vi "saveDataNodeBegin.vi"(8 "error in (no error)":errorcluster, 9 "indent":i32, 10 "XML Refnum in":refnum<file>, 11 "Channel in":refnum<class "Channel.lvclass">) -> (0 "error out":errorcluster, 2 "XML Refnum out":refnum<file>, 3 "Chennel out":refnum<class "Channel.lvclass">)   [LabVIEW 2014, in "Channel.lvclass"]
doc: "Begins the process of saving a xceData Node to an XML formatted file."
uses:
  Channel.lvclass
  Channel.lvclass/Channel.ctl
  xCE/xceDataNode/xceDataNode.lvclass
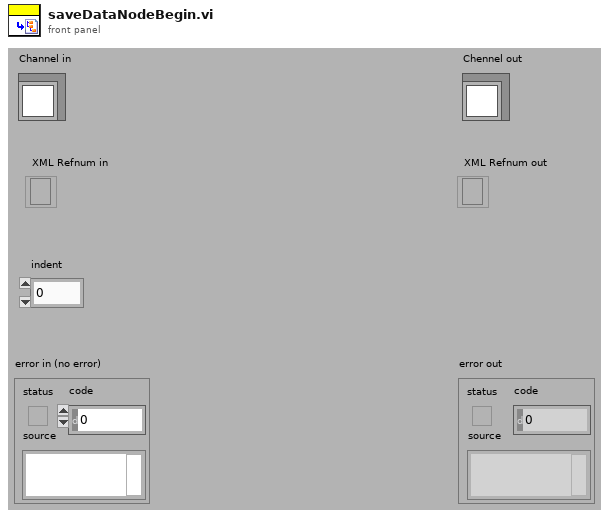
[diagram p1: front panel]
types:
  T1 = typedef "enum_Symbols.ctl" = enum16{"Default", "Analog Input", "Analog Output", "Digital Input", "Digital Output", "PWM Input", "PWM Output"}
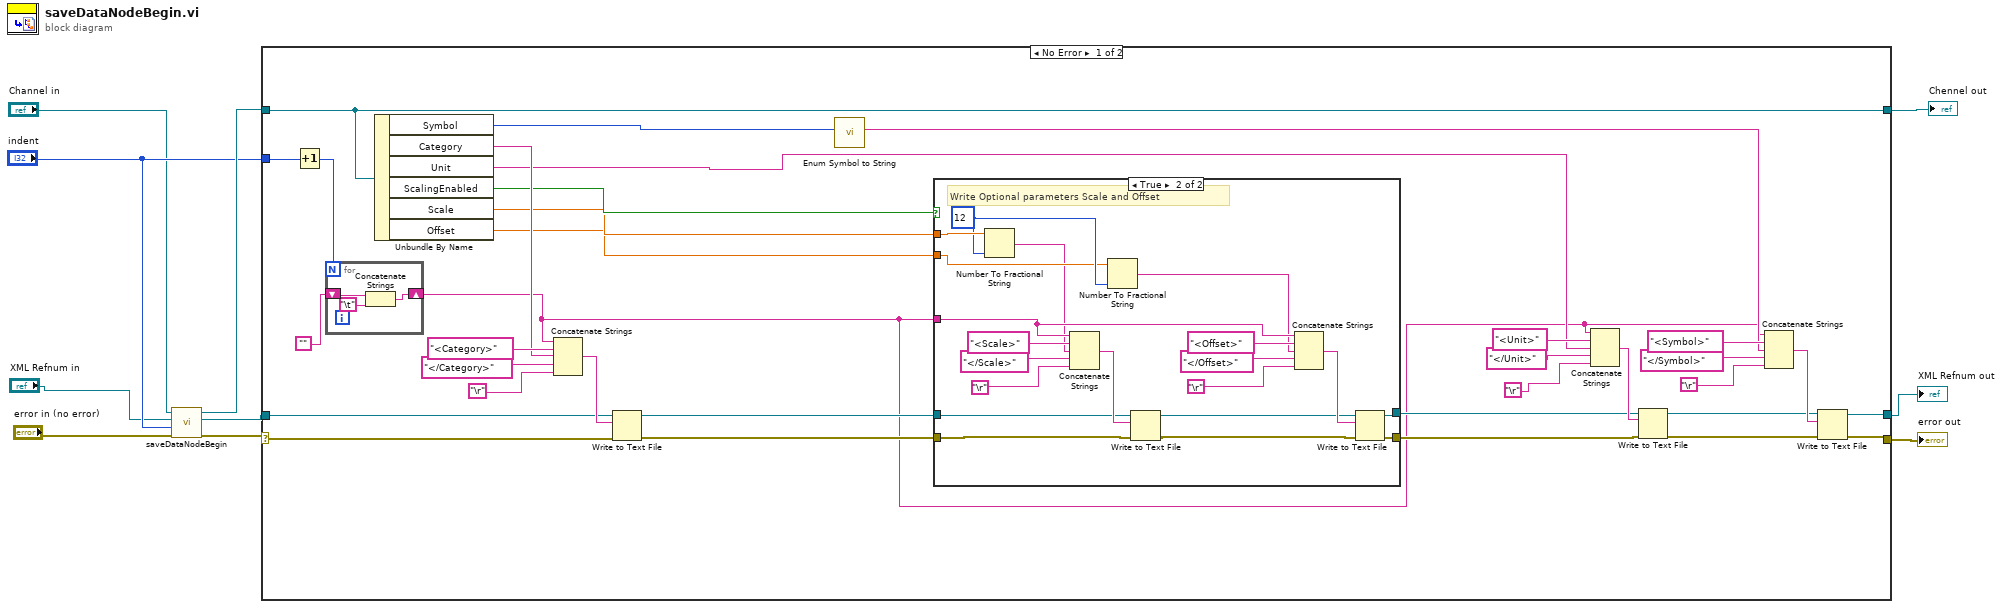
[diagram p0: block diagram]
diagram:
  n1 = call-parent "saveDataNodeBegin.vi"("error in (no error)"="error in (no error)", "indent"="indent", "XML Refnum in"="XML Refnum in", "xceDataNode in"="Channel in") -> ("error out"=w6:errorcluster, "XML Refnum out"=w5:refnum<file>, "xceDataNode out"=w4:refnum<class "Channel.lvclass">)  [unwired: 5 in]
  n2 = case shown="No Error" w6 {
    selector: w6 -> [w33 w71]
    tunnel: w4 -> [w35 w72]
    tunnel: [w35 w72] -> w10
    tunnel: [w12 w71] -> w8
    tunnel: [w13 w70] -> w9
    tunnel: "indent" -> [w36 _]
    tunnel: w5 -> [w34 w70]
    frame No Error {
      n3 = Increment(x=w36) -> (x+1=w43:i32)
      n4 = for {
        N: w43 -> [_]
        shift-right: [w67] -> w11
        shift-left: "" -> [w69]
        n5 = Concatenate Strings(w69, "\t") -> (w67:string)
      }
      n6 = Unbundle By Name(w35) -> ("Symbol"=w37:T1, "Category"=w38:string, "Unit"=w15:string, "ScalingEnabled"=w32:bool, "Scale"=w31:dbl, "Offset"=w30:dbl)
      n7 = Concatenate Strings(w11, "<Category>" ("string"), w38, "</Category>" ("string"), "\r") -> (w42:string)
      n8 = Write to Text File(file (use dialog)=w34, text=w42, error in=w33) -> (refnum out=w18:refnum<file>, error out=w17:errorcluster)  [unwired: 1 in, 1 out]
      n9 = call "Enum Symbol to String.vi"("Symbol Enum In"=w37) -> ("Symbol String Out"=w14:string)  [unwired: 10 in]
      n10 = case shown="True" w32 {
        tunnel: w18 -> [w46 w60]
        tunnel: w17 -> [w45 w59]
        tunnel: [w46 w47] -> w20
        tunnel: w11 -> [_ w57]
        tunnel: [w45 w54] -> w19
        tunnel: w31 -> [_ w53]
        tunnel: w30 -> [_ w51]
        frame False {
        }
        frame True {
          w52 = i16 12 ("precision (6)")
          # "Write Optional parameters Scale and Offset"
          n11 = Number To Fractional String(number=w53, precision (6)=w52) -> (F-format string=w50:string)  [unwired: 2 in]
          n12 = Concatenate Strings(w57, "<Scale>" ("string"), w50, "</Scale>" ("string"), "\r") -> (w66:string)
          n13 = Number To Fractional String(number=w51, precision (6)=w52) -> (F-format string=w49:string)  [unwired: 2 in]
          n14 = Write to Text File(file (use dialog)=w60, text=w66, error in=w59) -> (refnum out=w48:refnum<file>, error out=w58:errorcluster)  [unwired: 1 in, 1 out]
          n15 = Concatenate Strings(w57, "<Offset>" ("string"), w49, "</Offset>" ("string"), "\r") -> (w61:string)
          n16 = Write to Text File(file (use dialog)=w48, text=w61, error in=w58) -> (refnum out=w47:refnum<file>, error out=w54:errorcluster)  [unwired: 1 in, 1 out]
        }
      }
      n17 = Concatenate Strings(w11, "<Unit>" ("string"), w15, "</Unit>" ("string"), "\r") -> (w22:string)
      n18 = Write to Text File(file (use dialog)=w20, text=w22, error in=w19) -> (refnum out=w25:refnum<file>, error out=w21:errorcluster)  [unwired: 1 in, 1 out]
      n19 = Concatenate Strings(w11, "<Symbol>" ("string"), w14, "</Symbol>" ("string"), "\r") -> (w26:string)
      n20 = Write to Text File(file (use dialog)=w25, text=w26, error in=w21) -> (refnum out=w13:refnum<file>, error out=w12:errorcluster)  [unwired: 1 in, 1 out]
    }
    frame Error {
    }
  }
  "error out" <- w8
  "Chennel out" <- w10
  "XML Refnum out" <- w9
